vi "Read Image Dimensions.vi"(8 "error in (no error)":errorcluster, 11 "CCDCamera in":refnum<class "Simulated_CCD_Camera.lvclass">) -> (0 "error out":errorcluster, 2 "CCD Config":T1={"Exposure Time"=1.0, "Pre-amp gain"=0, "Readout Rate"=0, "EM Mode"=0, "EM Gain"=2, "Binning"=1, "Initial Line"=1, "Initial Cloumn"=1, "Final Line"=1024, "Final Column"=1024, "Kinetic Series Length"=1, "Shutter Mode"=2, "Cooler ON/OFF"=0, "Temperature"=0, "Image Name"="CH1", "Image Path"="C:\\Users\\observer\\Desktop\\Imagens", "Current Temperature"=20, "Temperatue Status"="TEMPERATURE OFF", "Serial Number"=9916, " #image"=0} {"Temperature" min=0 max=0; "EM Mode" items=["Electron Multiplying", "Conventional"]; "Readout Rate" items=["1 MHz", "10 MHz", "20 MHz", "30 MHz"]; "Pre-amp gain" items=["Gain 1", "Gain 2"]}, 3 "CCDCamera out":refnum<class "Simulated_CCD_Camera.lvclass">)   [LabVIEW 2018, in "Simulated_CCD_Camera.lvclass"]
uses:
  Simulated_CCD_Camera.lvclass
  Cooler/Cooler.lvclass
  C:/Users/observer/Desktop/SPARC4_ACS/Simulated_Cooler/Simulated_Cooler.lvclass
  Simulated_Cooler/Simulated_Cooler.lvclass
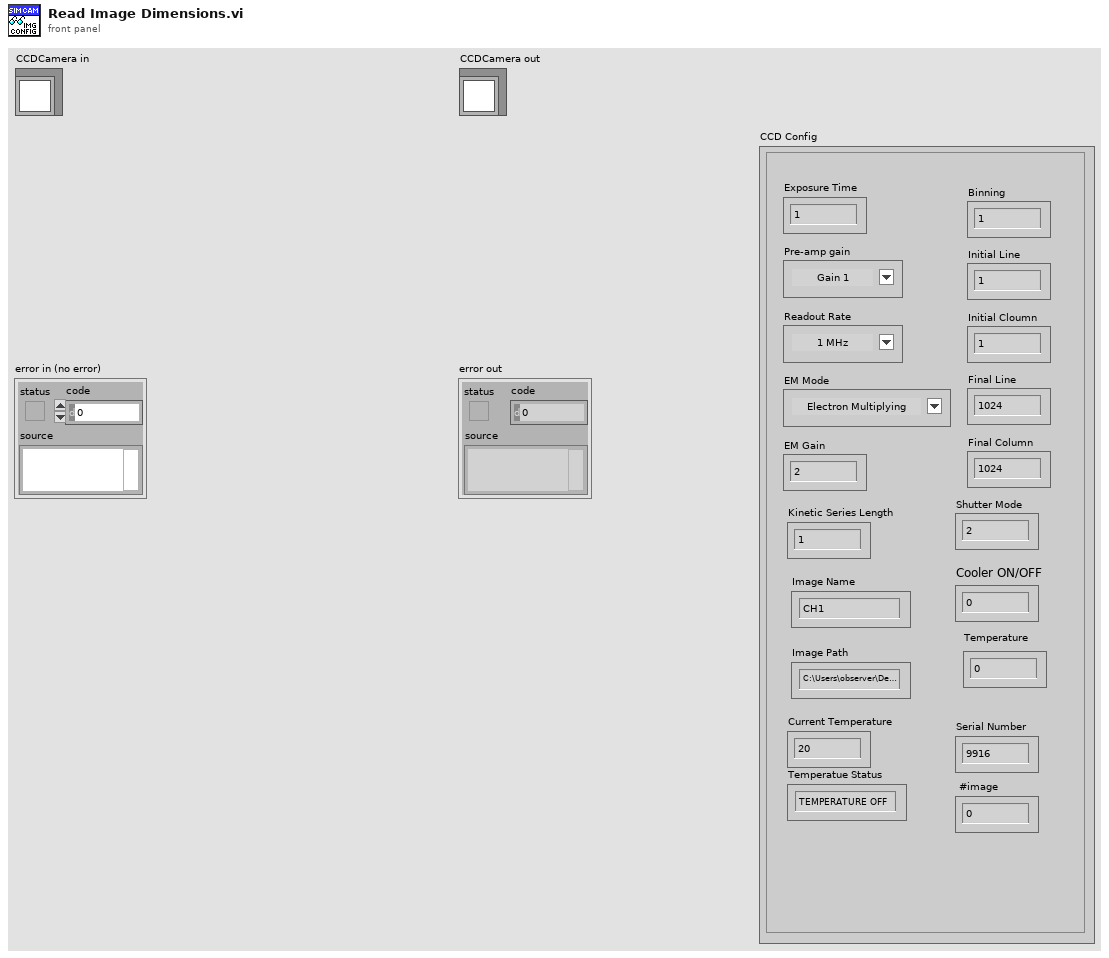
[diagram p1: front panel]
types:
  T1 = cluster{"Exposure Time":sgl, "Pre-amp gain":u8, "Readout Rate":u8, "EM Mode":u8, "EM Gain":u16, "Binning":u16, "Initial Line":u16, "Initial Cloumn":u16, "Final Line":u16, "Final Column":u16, "Kinetic Series Length":u32, "Shutter Mode":u8, "Cooler ON/OFF":u8, "Temperature":i8, "Image Name":string, "Image Path":string, "Current Temperature":i16, "Temperatue Status":string, "Serial Number":u16, " #image":u32}
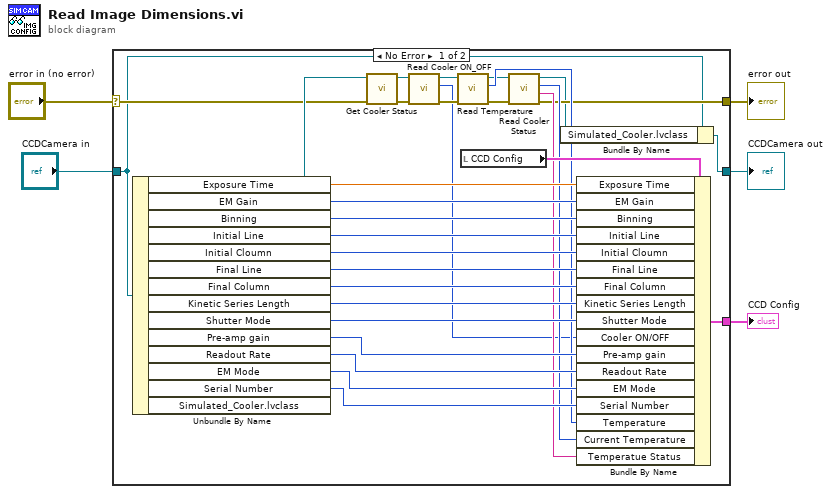
[diagram p0: block diagram]
diagram:
  n1 = case shown="No Error" "error in (no error)" {
    selector: "error in (no error)" -> [w20 w38]
    tunnel: [w14 w38] -> w4
    tunnel: [w11 w37] -> w2
    tunnel: "CCDCamera in" -> [w13 w37]
    tunnel: [w35 _] -> w1
    frame No Error {
      n2 = Unbundle By Name(w13) -> ("Exposure Time"=w23:sgl, "EM Gain"=w24:u16, "Binning"=w25:u16, "Initial Line"=w26:u16, "Initial Cloumn"=w27:u16, "Final Line"=w28:u16, "Final Column"=w29:u16, "Kinetic Series Length"=w30:u32, "Shutter Mode"=w22:u8, "Pre-amp gain"=w31:u8, "Readout Rate"=w32:u8, "EM Mode"=w33:u8, "Serial Number"=w34:u16, "Simulated_Cooler.lvclass"=w21:refnum<class "Simulated_Cooler.lvclass">)
      n3 = call "Get Cooler Status.vi"("error in (no error)"=w20, "Cooler in"=w21) -> ("error out"=w8:errorcluster, "Cooler out"=w9:refnum<class "Cooler.lvclass">)  [unwired: 8 in]
      n4 = call "Read Cooler ON_OFF.vi"("error in (no error)"=w8, "Cooler in"=w9) -> ("error out"=w7:errorcluster, "Cooler ON/OFF"=w6:u8, "Cooler out"=w10:refnum<class "Cooler.lvclass">)  [unwired: 7 in]
      n5 = call-dynamic "Read Temperature.vi"("error in (no error)"=w7, "Cooler in"=w10) -> ("error out"=w16:errorcluster, "Temperature"=w17:i32, "Cooler out"=w15:refnum<class "Cooler.lvclass">)  [unwired: 7 in]
      n6 = local read "CCD Config"() -> (w36:T1)
      n7 = call "Read Cooler Status.vi"("error in (no error)"=w16, "Cooler in"=w15) -> ("error out"=w14:errorcluster, "temp status"=w18:string, "Current temp"=w19:i16, "Cooler out"=w12:refnum<class "Cooler.lvclass">)  [unwired: 6 in]
      n8 = Bundle By Name(cluster=w13, "Simulated_Cooler.lvclass"=w12) -> (w11:refnum<class "Simulated_CCD_Camera.lvclass">)
      n9 = Bundle By Name(cluster=w36, "Exposure Time"=w23, "EM Gain"=w24, "Binning"=w25, "Initial Line"=w26, "Initial Cloumn"=w27, "Final Line"=w28, "Final Column"=w29, "Kinetic Series Length"=w30, "Shutter Mode"=w22, "Cooler ON/OFF"=w6, "Pre-amp gain"=w31, "Readout Rate"=w32, "EM Mode"=w33, "Serial Number"=w34, "Temperature"=w17, "Current Temperature"=w19, "Temperatue Status"=w18) -> (w35:T1)
    }
    frame Error {
    }
  }
  "error out" <- w4
  "CCDCamera out" <- w2
  "CCD Config" <- w1
